vi "center_particle_no_laser.vi"(0 "input_xyz":T3, 9 "parameters_xy-scan":T2={"image_size_xy_um"=1.0, "frame_size_xy_px"=10, "dwell_time_ms"=1.0} {"dwell_time_ms" format="%#_13g"; "image_size_xy_um" format="%#_13g"}, 11 "parameters_z-scan":T1={"dwell_time_ms"=10.0, "q_steps"=10, "span_um"=1.0, "refocus"=TRUE} {"dwell_time_ms" format="%#_13g"}) -> (4 "output_xyz":T3, 6 "mini_scan":dbl[][](array[numeric]))   [LabVIEW 2018]
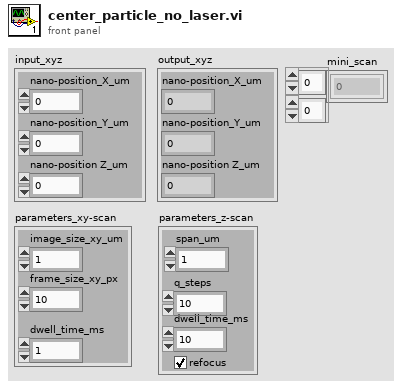
[diagram p1: front panel]
types:
  T1 = cluster{"dwell_time_ms":dbl, "q_steps":u32, "span_um":dbl, "refocus":bool}
  T2 = cluster{"image_size_xy_um":dbl, "frame_size_xy_px":u32, "dwell_time_ms":dbl}
  T3 = cluster{"nano-position_X_um":sgl, "nano-position_Y_um":sgl, "nano-position Z_um":sgl}
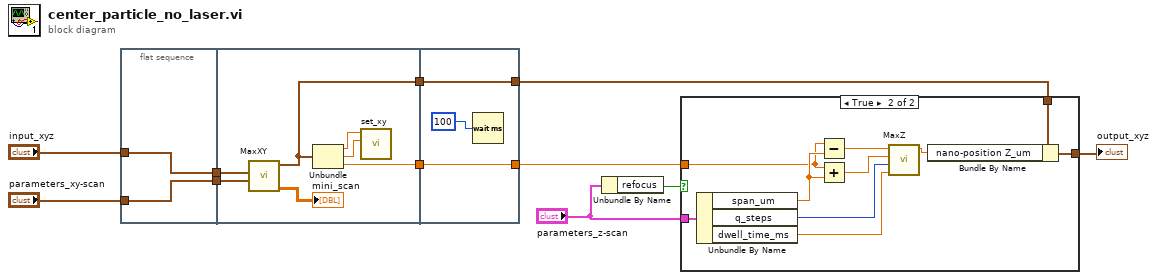
[diagram p0: block diagram]
diagram:
  n1 = flat-sequence {
    tunnel: "parameters_xy-scan" -> [w12]
    tunnel: "input_xyz" -> [w13]
    tunnel: [w13] -> w7
    tunnel: [w12] -> w6
    tunnel: [w15] -> w11
    tunnel: [w16] -> w9
    tunnel: w7 -> [w18]
    tunnel: w6 -> [w17]
    tunnel: w11 -> [w21]
    tunnel: w9 -> [w22]
    tunnel: [w22] -> w3
    tunnel: [w21] -> w2
    frame #0 {
    }
    frame #1 {
      n2 = call "MaxXY.vi"("input_xyz_um"=w18, "parameters_xy_scan"=w17) -> ("output_xyz_um"=w16:T3, "image"=→"mini_scan":dbl[][])  [unwired: 5 in, 2 out]
      n3 = Unbundle(w16) -> ("nano-position_X_um"=w19:sgl, "nano-position_Y_um"=w20:sgl, "nano-position Z_um"=w15:sgl)
      n4 = call "set_xy.vi"("y_value_um"=w20, "x_value_um"=w19) -> ()  [unwired: 9 in, 1 out]
    }
    frame #2 {
      n5 = Wait (ms)(milliseconds to wait=100) -> ()  [unwired: 1 out]
    }
  }
  n6 = Unbundle By Name("parameters_z-scan") -> ("refocus"=w5:bool)
  n7 = case shown="True" w5 {
    tunnel: w3 -> [w24 w34]
    tunnel: "parameters_z-scan" -> [_ w33]
    tunnel: [w24 w31] -> w1
    tunnel: w2 -> [_ w25]
    frame False {
    }
    frame True {
      n8 = Unbundle By Name(w33) -> ("span_um"=w32:dbl, "q_steps"=w27:u32, "dwell_time_ms"=w26:dbl)
      n9 = Subtract(x=w25, y=w32) -> (x-y=w29:dbl)
      n10 = Add(x=w25, y=w32) -> (x+y=w28:dbl)
      n11 = call "MaxZ.vi"("dwell_time_ms"=w26, "q_steps"=w27, "z_end_um"=w28, "z_start_um"=w29) -> ("z_focus_um"=w30:dbl)  [unwired: 6 in, 1 out]
      n12 = Bundle By Name(cluster=w34, "nano-position Z_um"=w30) -> (w31:T3)
    }
  }
  "output_xyz" <- w1
